vi "Host.vi"() -> ()   [LabVIEW 2018]
uses:
  <instrlib>/niDCPower/nidcpower.llb/niDCPower Measurement Type.ctl
panel:
  in  "Период опроса, мс":u32=1
  in  "Стоп":bool
  in  "Питание":bool
  in  "SEL_T, мс":u32=100
  in  "SIM_SEL":bool
  out "SEL":bool
  in  "5V на два канала_selcur":dbl=1.5 caption="current limit" format="%_6p"
  out "5V_cnt":i32
  out "5V_SEL":bool
  in  "5V, на два канала A":dbl=1.0 caption="current limit" format="%_6p"
  out "5V сумма_cur, A":dbl caption="measurement" format="%_6g"
  in  "5V, V":dbl=5.0 caption="voltage level" format="%_6p"
  out "5V_Chart":dbl(graph)=-0.03531418910399786
  in  "5V":refnum<k15>="PXI1Slot2" caption="instrument handle"
  in  "SEL":path=path "D:/VPL/24.100_VR очки"
  out "Номер образца":string="0"
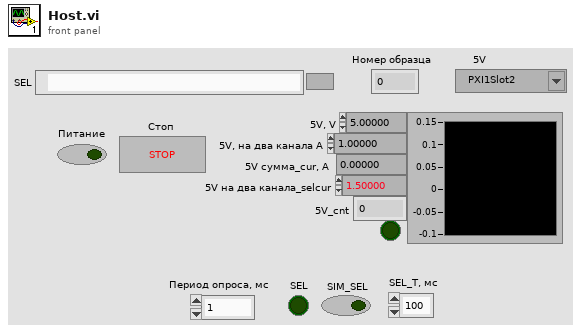
[diagram p1: front panel]
types:
  T1 = enum16{"open", "replace", "create", "open or create", "replace or create", "replace or create with confirmation"}
  T2 = typedef "niDCPower Measurement Type.ctl" = i32
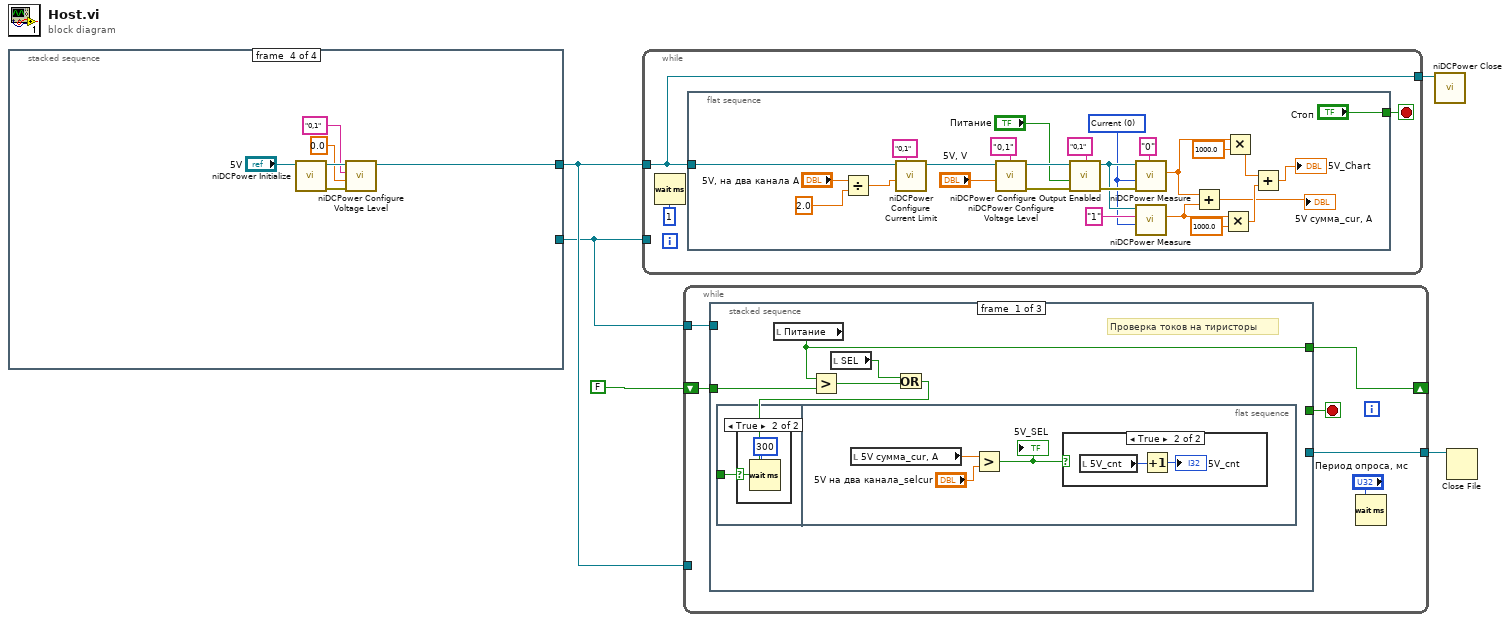
[diagram p0: block diagram]
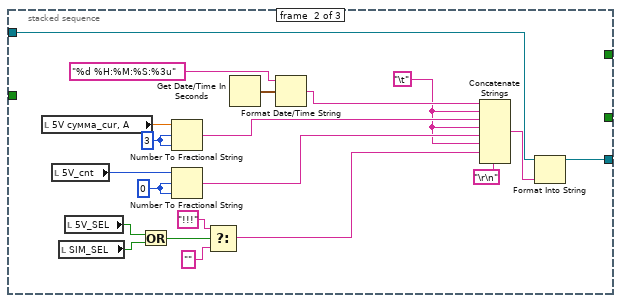
[diagram p4: hidden frame]
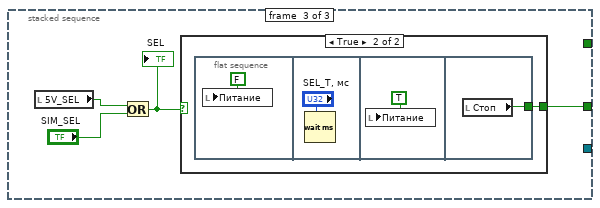
[diagram p5: hidden frame]
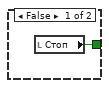
[diagram p6: hidden frame]
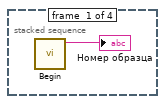
[diagram p7: hidden frame]
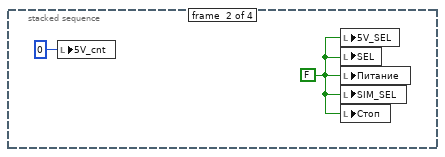
[diagram p8: hidden frame]
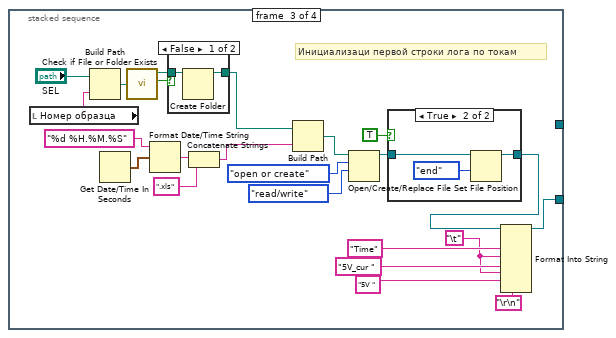
[diagram p9: hidden frame]
diagram:
  n1 = stacked-sequence {
    tunnel: [_ _ _ w39] -> w4
    tunnel: [_ _ w15 _] -> w3
    frame #0 {
      n2 = call "Begin.vi"() -> ("Номер образца 2"=→"Номер образца":string)  [unwired: 11 in]
    }
    frame #1 {
      w7 = FALSE
      n3 = local write "5V_cnt"(0) -> ()
      n4 = local write "5V_SEL"(w7) -> ()
      n5 = local write "SEL"(w7) -> ()
      n6 = local write "Питание"(w7) -> ()
      n7 = local write "SIM_SEL"(w7) -> ()
      n8 = local write "Стоп"(w7) -> ()
    }
    frame #2 {
      w11 = "\t"
      # "Инициализаци первой строки лога по токам"
      n9 = local read "Номер образца"() -> (w27:string)
      n10 = Build Path(base path="SEL", name or relative path=w27) -> (appended path=w29:path)
      n11 = Get Date/Time In Seconds() -> (seconds since 1Jan1904=w22:timestamp)
      n12 = call <vilib>:"Check if File or Folder Exists.vi"("path"=w29) -> ("file or folder exists?"=w30:bool, "dup path"=w31:path)  [unwired: 8 in, 1 out]
      n13 = Format Date/Time String(time format string (%c)="%d %H.%M.%S", seconds (now)=w22) -> (date/time string=w19:string)  [unwired: 1 in]
      n14 = case shown="False" w30 {
        tunnel: w31 -> [w37 w38]
        tunnel: [w36 w38] -> w14
        frame False {
          n15 = Create Folder(path (use dialog)=w37) -> (created path=w36:path)  [unwired: 2 in, 2 out]
        }
        frame True {
        }
      }
      n16 = Concatenate Strings(w19, ".xls" ("string")) -> (w17:string)
      n17 = Build Path(base path=w14, name or relative path=w17) -> (appended path=w20:path)
      n18 = Open/Create/Replace File(file path (use dialog)=w20, operation (0:open)=T1."open or create", access (0:read/write)=enum16{"read/write", "read-only", "write-only"}."read/write") -> (refnum out=w23:refnum<file>)  [unwired: 3 in, 2 out]
      n19 = case shown="True" TRUE {
        tunnel: w23 -> [w32 w35]
        tunnel: [w32 w33] -> w16
        frame False {
        }
        frame True {
          n20 = Set File Position(refnum=w35, from (0:start)=enum16{"start", "end", "current"}."end") -> (refnum out=w33:refnum<file>)  [unwired: 2 in, 1 out]
        }
      }
      n21 = Format Into String(initial string=w16, "Time" ("input 1"), w11, "5V_cur " ("input 1"), w11, "5V " ("input 1"), "\r\n") -> (resulting string=w15:refnum<file>)  [unwired: 2 in, 1 out]
    }
    frame #3 {
      n22 = call <instrlib>:"niDCPower Initialize.vi"("resource name"="5V") -> ("error out"=w43:errorcluster, "instrument handle out"=w44:refnum<k15>)  [unwired: 3 in, 6 out]
      n23 = call <instrlib>:"niDCPower Configure Voltage Level.vi"("error in (no error)"=w43, "voltage level"=0.0, "channel name"="0,1", "instrument handle"=w44) -> ("instrument handle out"=w39:refnum<k15>)  [unwired: 6 in, 1 out]
    }
  }
  n24 = while {
    tunnel: w4 -> [w45]
    tunnel: w3 -> [_]
    tunnel: [w45] -> w1
    stop <- w46 stop-if-true
    n25 = Wait (ms)(milliseconds to wait=u32 1) -> ()  [unwired: 1 out]
    n26 = flat-sequence {
      tunnel: w45 -> [w64]
      tunnel: ["Стоп"] -> w46
      frame #0 {
        w54 = T2 0 items=["Current", "Voltage"] ("measurement type")
        n27 = Divide(x="5V, на два канала A", y=2.0) -> (x/y=w48:dbl)
        n28 = call <instrlib>:"niDCPower Configure Current Limit.vi"("current limit"=w48, "channel name"="0,1", "instrument handle"=w64) -> ("instrument handle out"=w70:refnum<k15>)  [unwired: 7 in, 1 out]
        n29 = call <instrlib>:"niDCPower Configure Voltage Level.vi"("voltage level"="5V, V", "channel name"="0,1", "instrument handle"=w70) -> ("error out"=w67:errorcluster, "instrument handle out"=w68:refnum<k15>)  [unwired: 7 in]
        n30 = call <instrlib>:"niDCPower Configure Output Enabled.vi"("error in (no error)"=w67, "output enabled"="Питание", "channel name"="0,1", "instrument handle"=w68) -> ("error out"=w71:errorcluster, "instrument handle out"=w59:refnum<k15>)  [unwired: 6 in]
        n31 = call <instrlib>:"niDCPower Measure.vi"("error in (no error)"=w71, "measurement type"=w54, "channel name"="0", "instrument handle"=w59) -> ("measurement"=w53:dbl)  [unwired: 5 in, 2 out]
        n32 = call <instrlib>:"niDCPower Measure.vi"("measurement type"=w54, "channel name"="1", "instrument handle"=w59) -> ("measurement"=w52:dbl)  [unwired: 6 in, 2 out]
        n33 = Add(x=w53, y=w52) -> (x+y=→"5V сумма_cur, A":dbl)
        n34 = Multiply(x=w52, y=1000.0) -> (x*y=w56:dbl)
        n35 = Multiply(x=w53, y=1000.0) -> (x*y=w57:dbl)
        n36 = Add(x=w57, y=w56) -> (x+y=→"5V_Chart":dbl)
      }
    }
  }
  n37 = while {
    shift-right: [w79] -> _
    shift-left: FALSE -> [w78]
    tunnel: w3 -> [w77]
    tunnel: w4 -> [_]
    tunnel: [w75] -> w2
    stop <- w76 stop-if-true
    n38 = stacked-sequence {
      tunnel: [w83 _ _] -> w79
      tunnel: w78 -> [w84 _ _]
      tunnel: w77 -> [_ w105 _]
      tunnel: [_ _ w115] -> w76
      tunnel: [_ w100 _] -> w75
      frame #0 {
        # "Проверка токов на тиристоры"
        n39 = flat-sequence {
          tunnel: w80 -> [w85]
          frame #0 {
            n40 = case shown="True" w85 {
              frame False {
              }
              frame True {
                n41 = Wait (ms)(milliseconds to wait=u32 300) -> ()  [unwired: 1 out]
              }
            }
          }
          frame #1 {
            n42 = local read "5V сумма_cur, A"() -> (w87:dbl)
            n43 = Greater?(x=w87, y="5V на два канала_selcur") -> (0:w88:bool)
            "5V_SEL" <- w88
            n44 = case shown="True" w88 {
              frame False {
              }
              frame True {
                n45 = local read "5V_cnt"() -> (w91:i32)
                n46 = Increment(x=w91) -> (x+1=→"5V_cnt":i32)
              }
            }
          }
        }
        n47 = local read "Питание"() -> (w83:bool)
        n48 = Greater?(x=w83, y=w84) -> (0:w82:bool)
        n49 = local read "SEL"() -> (w81:bool)
        n50 = Or(x=w81, y=w82) -> (x .or. y?=w80:bool)
      }
      frame #1 {
        w103 = i16 0 ("width (-)")
        w102 = i16 3 ("width (-)")
        w94 = "\t"
        n51 = local read "5V сумма_cur, A"() -> (w104:dbl)
        n52 = local read "5V_cnt"() -> (w101:i32)
        n53 = local read "SIM_SEL"() -> (w97:bool)
        n54 = local read "5V_SEL"() -> (w99:bool)
        n55 = Or(x=w99, y=w97) -> (x .or. y?=w98:bool)
        n56 = Number To Fractional String(number=w104, width (-)=w102, precision (6)=w102) -> (F-format string=w96:string)  [unwired: 1 in]
        n57 = Number To Fractional String(number=w101, width (-)=w103, precision (6)=w103) -> (F-format string=w95:string)  [unwired: 1 in]
        n58 = Select(t="!!!", s=w98, f="") -> (s? t:f=w93:string)
        n59 = Get Date/Time In Seconds() -> (seconds since 1Jan1904=w111:timestamp)
        n60 = Format Date/Time String(time format string (%c)="%d %H:%M:%S:%3u", seconds (now)=w111) -> (date/time string=w106:string)  [unwired: 1 in]
        n61 = Concatenate Strings(w106, w94, w96, w94, w95, w94, w93, "\r\n") -> (w110:string)
        n62 = Format Into String(initial string=w105, w110) -> (resulting string=w100:refnum<file>)  [unwired: 2 in, 1 out]
      }
      frame #2 {
        n63 = local read "5V_SEL"() -> (w113:bool)
        n64 = Or(x=w113, y="SIM_SEL") -> (x .or. y?=w114:bool)
        "SEL" <- w114
        n65 = case shown="True" w114 {
          tunnel: [w116 w117] -> w115
          frame False {
            n66 = local read "Стоп"() -> (w116:bool)
          }
          frame True {
            n67 = flat-sequence {
              tunnel: [w121] -> w117
              frame #0 {
                n68 = local write "Питание"(FALSE ("SYS_RESET")) -> ()
              }
              frame #1 {
                n69 = Wait (ms)(milliseconds to wait="SEL_T, мс") -> ()  [unwired: 1 out]
              }
              frame #2 {
                n70 = local write "Питание"(TRUE ("SYS_RESET")) -> ()
              }
              frame #3 {
                n71 = local read "Стоп"() -> (w121:bool)
              }
            }
          }
        }
      }
    }
    n72 = Wait (ms)(milliseconds to wait="Период опроса, мс") -> ()  [unwired: 1 out]
  }
  n73 = call <instrlib>:"niDCPower Close.vi"("instrument handle"=w1) -> ()  [unwired: 10 in, 1 out]
  n74 = Close File(refnum=w2) -> ()  [unwired: 1 in, 2 out]
